vi "WriteToINIFile.vi"(8 "error in (no error)":errorcluster, 10 "Refnum in":T1, 11 "RoomAlert in":refnum<class "RoomAlert.lvclass">) -> (0 "error out":errorcluster, 3 "RoomAlert out":refnum<class "RoomAlert.lvclass">)   [LabVIEW 2018, in "SensorPlugins.lvlib" / "RoomAlert.lvclass"]
uses:
  RoomAlert.lvclass
  <vilib>/Utility/config.llb/Config Data RefNum.ctl
  <vilib>/Utility/config.llb/NI_LVConfig.lvlib
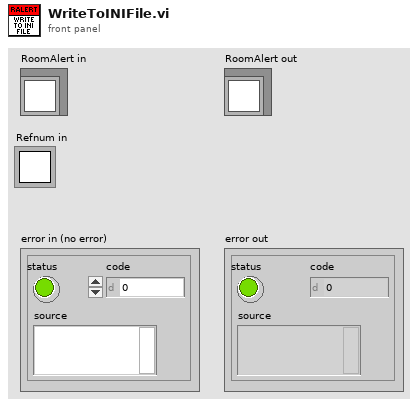
[diagram p1: front panel]
types:
  T1 = typedef "NI_LVConfig.lvlib/Config Data RefNum.ctl" = refnum<k1>
  T2 = typedef "SensorPlugins.lvlib/RoomAlert.lvclass/RoomAlertControls.ctl" = cluster{"Connected?":bool, "IP Address of SNMP Device":string, "Port (502)":u16, "GET OID ARRAY":string[], "SET OID ARRAY":string[][], "Community Name":string, "Measurements To Read Array":u16[], "Use Measurement To Read Array":bool}[]
  T3 = typedef "SensorPlugins.lvlib/RoomAlert.lvclass/MeasurementControls.ctl" = cluster{"Measurement RefreshTime (ms)":u32, "Measurement Name":string, "Timeout(ms)":i32}
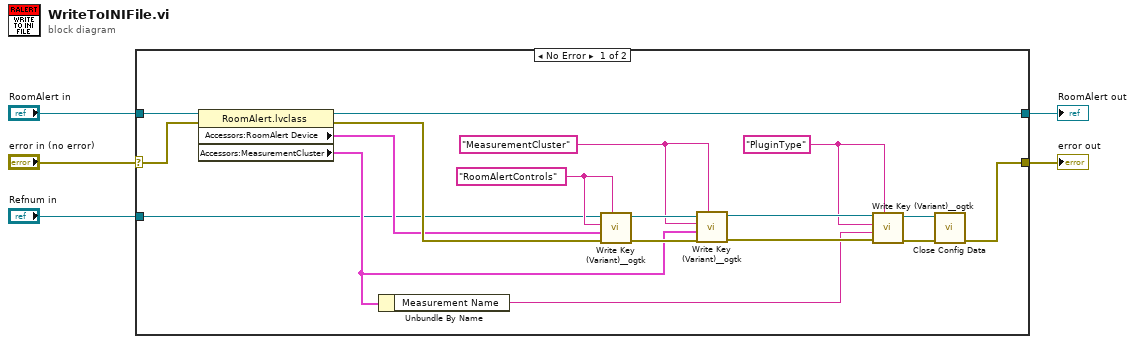
[diagram p0: block diagram]
diagram:
  n1 = case shown="No Error" "error in (no error)" {
    selector: "error in (no error)" -> [w21 w25]
    tunnel: "RoomAlert in" -> [w22 w24]
    tunnel: [w20 w24] -> w2
    tunnel: [w17 w25] -> w3
    tunnel: "Refnum in" -> [w6 _]
    frame No Error {
      w8 = "PluginType" ("section (optional)")
      w14 = "MeasurementCluster" ("section (optional)")
      w23 = "RoomAlertControls" ("section (optional)")
      n2 = property class="RoomAlert.lvclass"(reference=w22, error in=w21) -> (reference out=w20:refnum<class "RoomAlert.lvclass">, error out=w19:errorcluster, "Accessors:RoomAlert Device"=w18:T2, "Accessors:MeasurementCluster"=w7:T3)
      n3 = Unbundle By Name(w7) -> ("Measurement Name"=w9:string)
      n4 = call <userlib>:"Write Key (Variant)__ogtk.vi"("section"=w23, "error in (no error)"=w19, "key-value"=w18, "key (optional)"=w23, "refnum"=w6) -> ("error out"=w16:errorcluster, "refnum out"=w15:T1)  [unwired: 5 in]
      n5 = call <userlib>:"Write Key (Variant)__ogtk.vi"("section"=w14, "error in (no error)"=w16, "key-value"=w7, "key (optional)"=w14, "refnum"=w15) -> ("error out"=w13:errorcluster, "refnum out"=w12:T1)  [unwired: 5 in]
      n6 = call <userlib>:"Write Key (Variant)__ogtk.vi"("section"=w8, "error in (no error)"=w13, "key-value"=w9, "key (optional)"=w8, "refnum"=w12) -> ("error out"=w11:errorcluster, "refnum out"=w10:T1)  [unwired: 5 in]
      n7 = call <vilib>:"Close Config Data.vi"("error in (no error)"=w11, "refnum"=w10) -> ("error out"=w17:errorcluster)  [unwired: 8 in, 1 out]
    }
    frame Error {
    }
  }
  "error out" <- w3
  "RoomAlert out" <- w2
